vi "Get IP address and hostname.vi"(8 "error in (no error)":errorcluster, 10 "Hostname In":string, 11 "IP Address In":string) -> (0 "error out":errorcluster, 2 "Found Hostname":string, 3 "Found IP":string)   [LabVIEW 2024, in "Session Scanner.lvlib"]
uses:
  Session Scanner.lvlib
  <vilib>/Utility/error.llb/Trim Whitespace One-Sided.vi
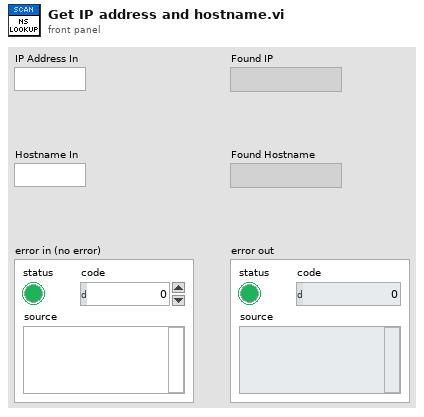
[diagram p1: front panel]
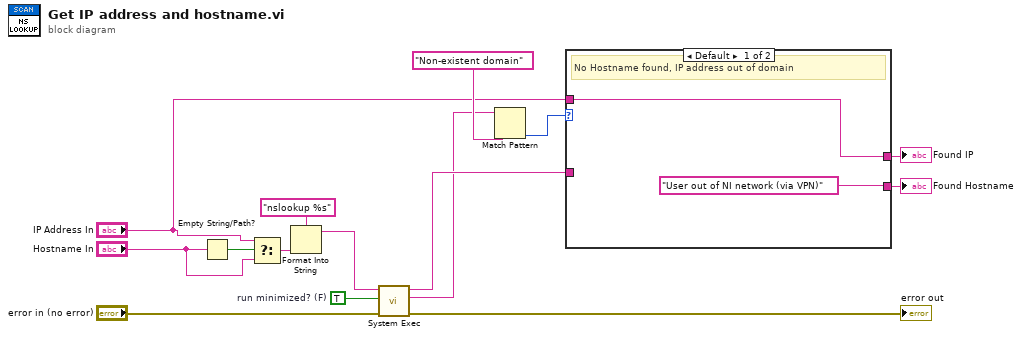
[diagram p0: block diagram]
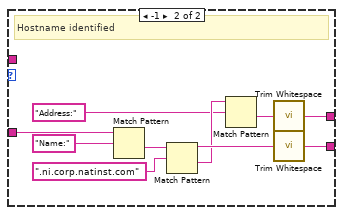
[diagram p2: hidden frame]
diagram:
  w10 = TRUE  # run minimized? (F)
  n1 = Empty String/Path?(string/path="Hostname In") -> (empty?=w13:bool)
  n2 = Select(t="IP Address In", s=w13, f="Hostname In") -> (s? t:f=w9:string)
  n3 = Format Into String(format string="nslookup %s", w9) -> (resulting string=w12:string)  [unwired: 2 in, 1 out]
  n4 = call <vilib>:"System Exec.vi"("run minimized? (F)"=w10, "error in (no error)"="error in (no error)", "command line"=w12) -> ("error out"=→"error out":errorcluster, "standard error"=w1:string, "standard output"=w5:string)  [unwired: 5 in, 1 out]
  n5 = Match Pattern(string=w1, regular expression="Non-existent domain") -> (offset past match=w3:i32)  [unwired: 1 in, 3 out]
  n6 = case shown="Default" w3 {
    tunnel: w5 -> [_ w25]
    tunnel: [w17 w19] -> w7
    tunnel: ["User out of NI network (via VPN)" ("trimmed string") w18] -> w6
    tunnel: "IP Address In" -> [w17 _]
    frame Default {
      # "No Hostname found, IP address out of domain"
    }
    frame -1 {
      # "Hostname identified"
      n7 = Match Pattern(string=w25, regular expression="Name:") -> (after substring=w26:string)  [unwired: 1 in, 3 out]
      n8 = Match Pattern(string=w26, regular expression=".ni.corp.natinst.com") -> (before substring=w27:string, after substring=w23:string)  [unwired: 1 in, 2 out]
      n9 = Match Pattern(string=w23, regular expression="Address:") -> (after substring=w24:string)  [unwired: 1 in, 3 out]
      n10 = call <vilib>:"Trim Whitespace.vi"("string"=w24) -> ("trimmed string"=w19:string)  [unwired: 1 in]
      n11 = call <vilib>:"Trim Whitespace.vi"("string"=w27) -> ("trimmed string"=w18:string)  [unwired: 1 in]
    }
  }
  "Found IP" <- w7
  "Found Hostname" <- w6
